vi "Bus Interface.vi"(0 "DIO":refnum<class "Digital IO.lvclass">, 1 "abort":bool, 5 "instruction":T2, 9 "input valid":bool) -> (6 "response":T1, 10 "done":bool, 14 "ready for input":bool)   [LabVIEW 2017, in "Digital IO.lvlib" / "Digital IO.lvclass"]
uses:
  Digital IO.lvclass
  <instrlib>/_niInstr/Instruction Framework/v1/FPGA/Interfaces/Address Space/Address Space Instruction.ctl
  <instrlib>/_niInstr/Instruction Framework/v1/FPGA/Typedefs/Response.ctl
  <instrlib>/_niInstr/Instruction Framework/v1/FPGA/Typedefs/niInstr Instruction Framework v1 FPGA.lvlib
  <instrlib>/_niInstr/Instruction Framework/v1/FPGA/Interfaces/Address Space/Address Space.lvclass
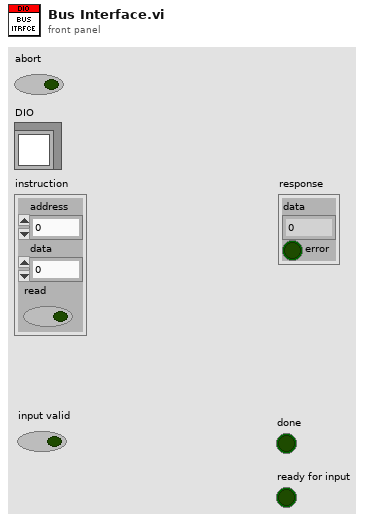
[diagram p1: front panel]
types:
  T1 = typedef "niInstr Instruction Framework v1 FPGA.lvlib/Response.ctl" = cluster{"data":u64, "error":bool}
  T2 = typedef "niInstr Instruction Framework Interfaces v1 FPGA.lvlib/Address Space.lvclass/Address Space Instruction.ctl" = cluster{"address":u32, "data":u64, "read":bool}
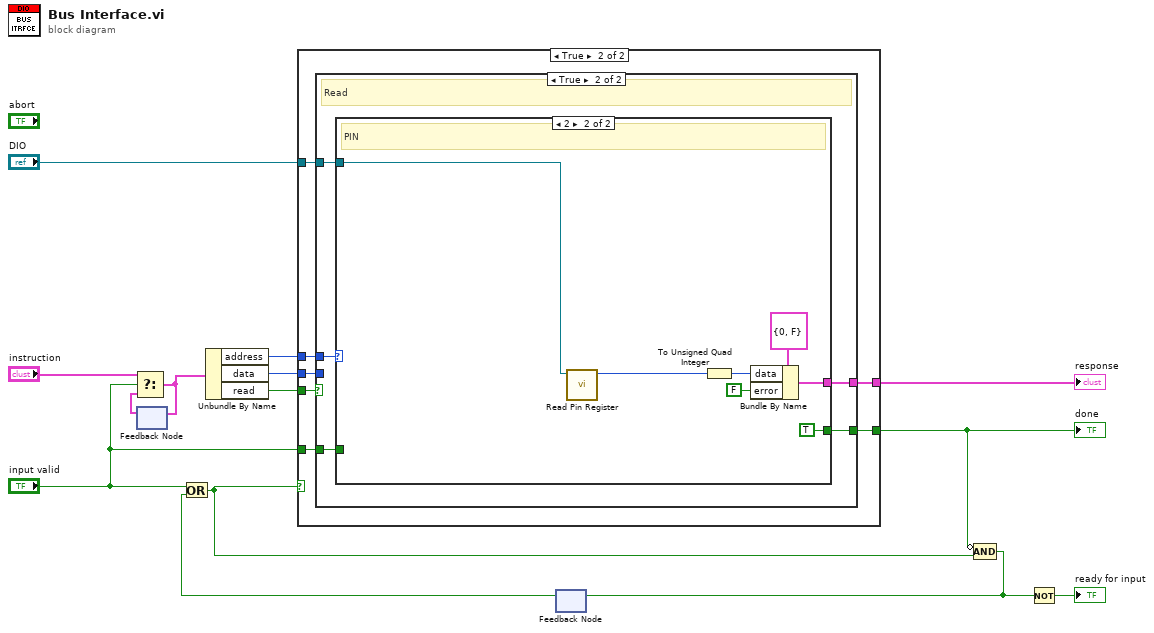
[diagram p0: block diagram]
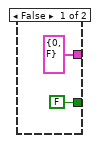
[diagram p2: hidden frame]
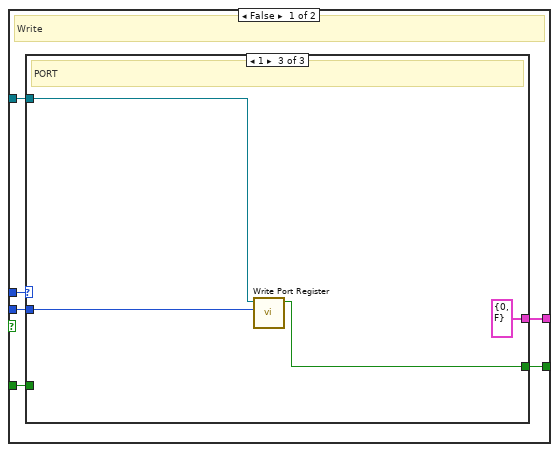
[diagram p3: hidden frame]
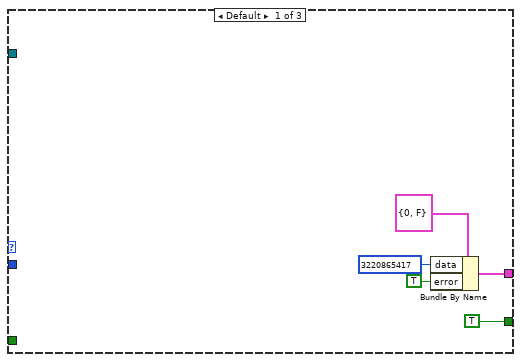
[diagram p4: hidden frame]
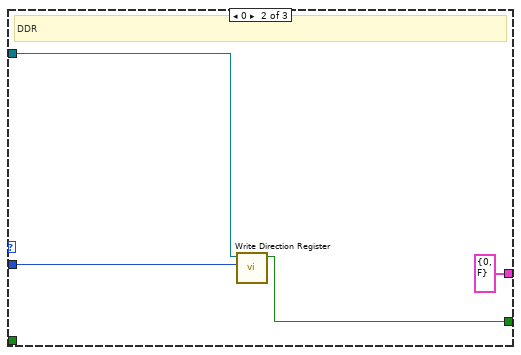
[diagram p5: hidden frame]
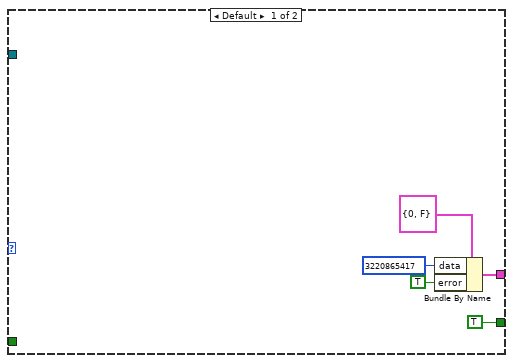
[diagram p6: hidden frame]
diagram:
  n1 = feedback #1() -> (w13:T2)  [unwired: 1 in]
  n2 = Select(t="instruction", s="input valid", f=w13) -> (s? t:f=w12:T2)
  n3 = feedback-in #1(w12) -> ()
  n4 = Unbundle By Name(w12) -> ("address"=w9:u32, "data"=w10:u64, "read"=w11:bool)
  n5 = feedback #2() -> (w3:bool)  [unwired: 1 in]
  n6 = Or(x="input valid", y=w3) -> (x .or. y?=w4:bool)
  n7 = case shown="True" w4 {
    tunnel: w11 -> [_ w23]
    tunnel: w9 -> [_ w22]
    tunnel: w10 -> [_ w21]
    tunnel: [T1 {"data"=0, "error"=FALSE} ("response") w20] -> w8
    tunnel: [FALSE ("Output Valid") w19] -> w1
    tunnel: "DIO" -> [_ w18]
    tunnel: "input valid" -> [_ w17]
    frame False {
    }
    frame True {
      n8 = case shown="True" w23 {
        tunnel: w22 -> [w29 w47]
        tunnel: w21 -> [w28 _]
        tunnel: [w27 w46] -> w20
        tunnel: [w26 w45] -> w19
        tunnel: w18 -> [w25 w44]
        tunnel: w17 -> [w24 w43]
        frame False {
          # "Write"
          n9 = case shown="1" w29 {
            tunnel: w28 -> [_ w38 w42]
            tunnel: [w31 T1 {"data"=0, "error"=FALSE} ("response") T1 {"data"=0, "error"=FALSE} ("response")] -> w27
            tunnel: [TRUE ("done") w36 w40] -> w26
            tunnel: w25 -> [_ w37 w41]
            tunnel: w24 -> [_ _ _]
            frame Default {
              n10 = Bundle By Name(cluster=T1 {"data"=0, "error"=FALSE} ("response"), "data"=u64 3220865417, "error"=TRUE) -> (w31:T1)
            }
            frame 0 {
              # "DDR"
              n11 = call-dynamic "Write Direction Register.vi"("data"=w38, "GPIO in"=w37) -> ("done"=w36:bool)  [unwired: 9 in]
            }
            frame 1 {
              # "PORT"
              n12 = call-dynamic "Write Port Register.vi"("data"=w42, "GPIO in"=w41) -> ("done"=w40:bool)  [unwired: 9 in]
            }
          }
        }
        frame True {
          # "Read"
          n13 = case shown="2" w47 {
            tunnel: [w49 w56] -> w46
            tunnel: [TRUE ("done") TRUE ("done")] -> w45
            tunnel: w44 -> [_ w59]
            tunnel: w43 -> [_ _]
            frame Default {
              n14 = Bundle By Name(cluster=T1 {"data"=0, "error"=FALSE} ("response"), "data"=u64 3220865417, "error"=TRUE) -> (w49:T1)
            }
            frame 2 {
              # "PIN"
              n15 = call-dynamic "Read Pin Register.vi"("GPIO in"=w59) -> ("pin register"=w55:u8)  [unwired: 10 in]
              n16 = To Unsigned Quad Integer(1:w55) -> (0:w54:u64)
              n17 = Bundle By Name(cluster=T1 {"data"=0, "error"=FALSE} ("response"), "data"=w54, "error"=FALSE) -> (w56:T1)
            }
          }
        }
      }
    }
  }
  "done" <- w1
  "response" <- w8
  n18 = Compound Arithmetic op=AND(invert w1, w4) -> (w5:bool)
  n19 = feedback-in #2(w5) -> ()
  n20 = Not(x=w5) -> (.not. x?=→"ready for input":bool)
